vi "Overlay Text.vi"(8 "error in (no error)":errorcluster, 10 "Pixel Coordinates":cluster{"X":dbl, "Y":dbl}[](array[cluster]), 11 "Refnum in":T1) -> (0 "error out":errorcluster)   [LabVIEW 2020]
uses:
  <vilib>/vision/Image Controls.llb/IMAQ Image.ctl
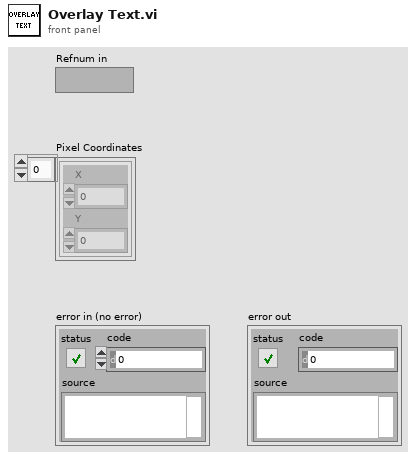
[diagram p1: front panel]
types:
  T1 = typedef "IMAQ Image.ctl" = refnum<image>
  T2 = cluster{"Desired Font (Application)":enum16{"User-specified Font", "Application Font", "System Font", "Dialog Font"}, "[User-specified Font]":cluster{"Font Name":string, "Size":i16, "Strikeout?":bool, "Italic?":bool, "Underline?":bool, "Outline?":bool, "Shadow?":bool, "Bold?":bool, "Rotation Angle":dbl}, "Horizontal Alignment":i16, "Vertical Alignment":i16}
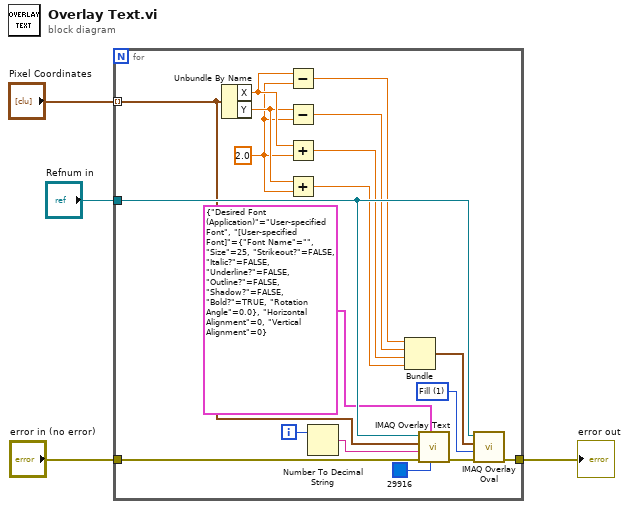
[diagram p0: block diagram]
diagram:
  n1 = for {
    tunnel: "Refnum in" -> [w22]
    tunnel: "error in (no error)" -> [w16]
    tunnel: [w6] -> w2
    tunnel: "Pixel Coordinates" -> [w5] mode=indexing
    i -> [w21]
    w7 = u32 1 items=["Frame", "Fill"] ("Drawing Mode (Frame)")
    w17 = 2.0 ("Y")
    n2 = Unbundle By Name(w5) -> ("X"=w19:dbl, "Y"=w18:dbl)
    n3 = Subtract(x=w19, y=w17) -> (x-y=w14:dbl)
    n4 = Subtract(x=w18, y=w17) -> (x-y=w13:dbl)
    n5 = Add(x=w19, y=w17) -> (x+y=w12:dbl)
    n6 = Add(x=w18, y=w17) -> (x+y=w11:dbl)
    n7 = Number To Decimal String(number=w21) -> (decimal integer string=w20:string)  [unwired: 1 in]
    n8 = Bundle(w14, w13, w12, w11) -> (w10:cluster{dbl, dbl, dbl, dbl})  [unwired: 1 in]
    n9 = call "IMAQ Overlay Text"("Text Color (black)"=u32 29916, "Font, Size & Style"=T2 {"Desired Font (Application)"=enum."User-specified Font", "[User-specified Font]"={"Font Name"="", "Size"=25, "Strikeout?"=FALSE, "Italic?"=FALSE, "Underline?"=FALSE, "Outline?"=FALSE, "Shadow?"=FALSE, "Bold?"=TRUE, "Rotation Angle"=0.0}, "Horizontal Alignment"=0, "Vertical Alignment"=0}, "error in (no error)"=w16, "String"=w20, "Origin"=w5, "Image"=w22) -> ("error out"=w15:errorcluster)  [unwired: 4 in, 1 out]
    n10 = call "IMAQ Overlay Oval"("error in (no error)"=w15, "Drawing Mode (Frame)"=w7, "Bounding Rectangle"=w10, "Image"=w22) -> ("error out"=w6:errorcluster)  [unwired: 6 in, 1 out]
  }
  "error out" <- w2
